vi "Zernike Array SLM.vi"() -> (8 "zernike array":dbl[][][](array[numeric]))   [LabVIEW 2014]
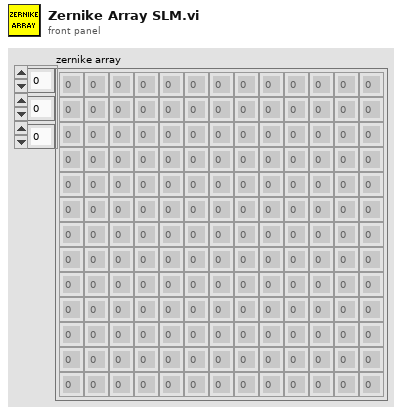
[diagram p1: front panel]
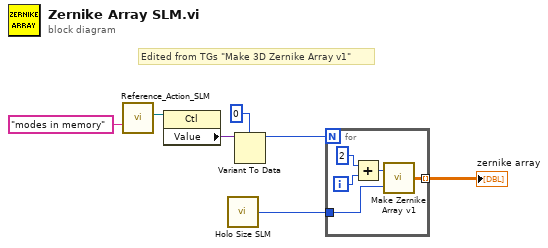
[diagram p0: block diagram]
diagram:
  # "Edited from TGs \"Make 3D Zernike Array v1\""
  n1 = call "Reference_Action_SLM.vi"("Control Name"="modes in memory") -> ("Ref OUT"=w4:refnum<vi>)  [unwired: 12 in, 2 out]
  n2 = property class="Ctl"(reference=w4) -> ("Value"=w5:variant)  [unwired: 1 in, 2 out]
  n3 = call "Holo Size SLM.vi"() -> ("data"=w1:i32)  [unwired: 15 in]
  n4 = Variant To Data(type=0, Variant=w5) -> (data=w7:i32)  [unwired: 1 in, 1 out]
  n5 = for {
    N: w7 -> [_]
    tunnel: w1 -> [w12]
    tunnel: [w8] -> w2 mode=indexing
    i -> [w10]
    n6 = Add(x=2, y=w10) -> (x+y=w11:i32)
    n7 = call "Make Zernike Array v1.vi"("size"=w12, "z"=w11) -> ("zernike array"=w8:dbl[][])
  }
  "zernike array" <- w2
